vi "Uni final.vi"() -> ()   [LabVIEW 2025]
uses:
  <vilib>/MakerHub/LINX/Public/Peripherals/Analog/Analog Read 1 Chan.vi
  <vilib>/MakerHub/LINX/Public/Peripherals/Analog/Analog Read N Chans.vi
  <vilib>/MakerHub/LINX/Private/Local IO/LinxAnalogRead.vi
  <vilib>/MakerHub/LINX/Public/Utilities/Check Channel.vi
  <vilib>/MakerHub/LINX/Public/Utilities/Open Serial.vi
  <vilib>/MakerHub/LINX/Private/Utilties/Generate Error.vi
  <vilib>/MakerHub/LINX/LMH-LINX.lvlib
panel:
  out "Presión de Frenado":dbl(knob) scale=0.0..1000.0
  out "COLD":bool
  out "HOT":bool
  out "Presion de Frenado":dynamicdata(graph)
  out "Termometro K":dbl(slide) scale=0.0..400.0
  out "Termometro F":dbl(slide) scale=0.0..160.0
  out "Batería Descargada":bool
  out "Batería Cargada":bool
  in  "Serial Port":refnum<visa-resource-name>="N/A"
  in  "Stop":bool
  out "RPM":dbl(knob) scale=0.0..7000.0
  out "Batería":dbl(slide) scale=0.0..100.0
  out "Teermometro °C":dbl(slide) scale=0.0..170.0
  # "Universidad Politécnica Salesiana"
  # "PROYECTO 1"
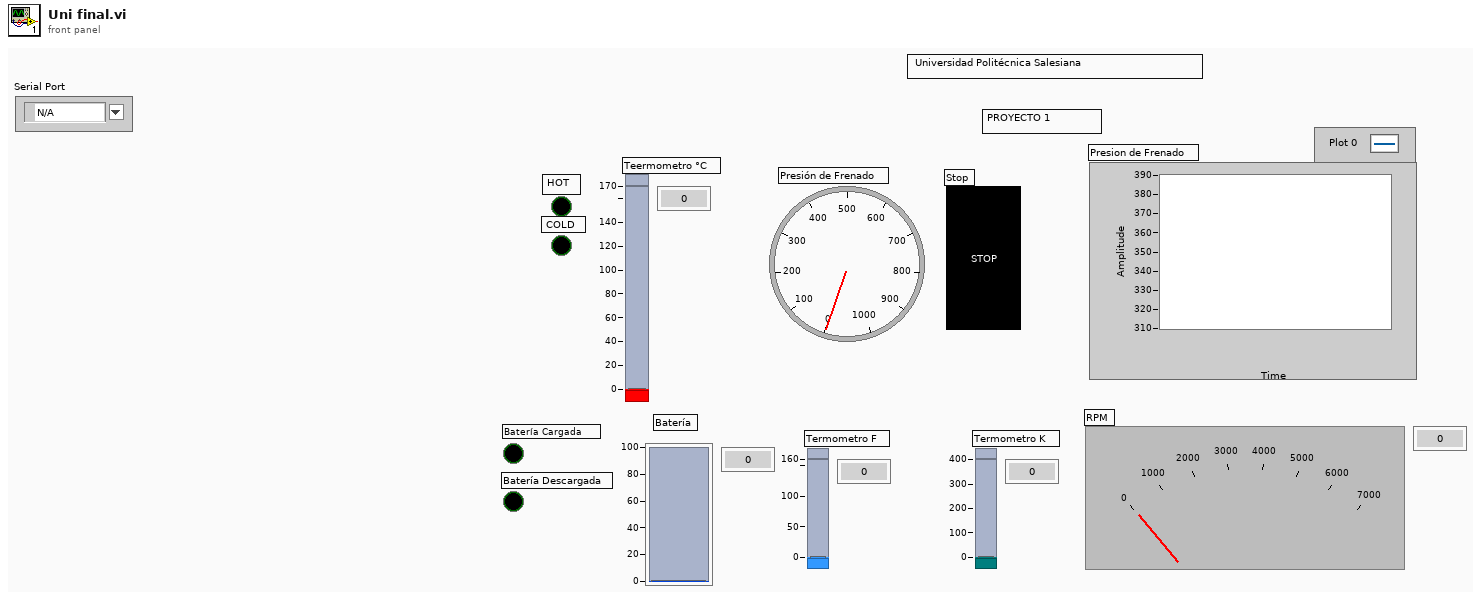
[diagram p1: front panel]
types:
  T1 = typedef "LMH-LINX.lvlib/LINX Ref.ctl" = cluster{"IO":T2, "Interface":T3, "LINX Device Config":T4}
  T2 = typedef "LMH-LINX.lvlib/Platform.ctl" = enum16{"Remote", "Local"}
  T3 = typedef "LMH-LINX.lvlib/Interface.ctl" = enum16{"Serial", "TCP"}
  T4 = typedef "LMH-LINX.lvlib/Device.lvlib/LINX Device Config.ctl" = cluster{"Interface":T3, "COM Port":refnum<visa-resource-name>, "TCP Configuration":T5, "Device Family":u8, "Device ID":u8, "Device Name":string, "TCP Ref":refnum<k5>, "Channels":T6}
  T5 = typedef "LMH-LINX.lvlib/Device.lvlib/TCP Config.ctl" = cluster{"IP Address":string, "Port":u16}
  T6 = typedef "LMH-LINX.lvlib/Channels.ctl" = cluster{"DI":u8[], "DO":u8[], "AI":u8[], "AO":u8[], "PWM":u8[], "QE":u8[], "UART":u8[], "I2C 2":u8[], "SPI":u8[], "CAN":u8[], "Servo":u8[], "AI Ref (V)":dbl, "AI Resolution (Bits)":u8, "AO Ref (V)":dbl, "AO Resolution (Bits)":u8}
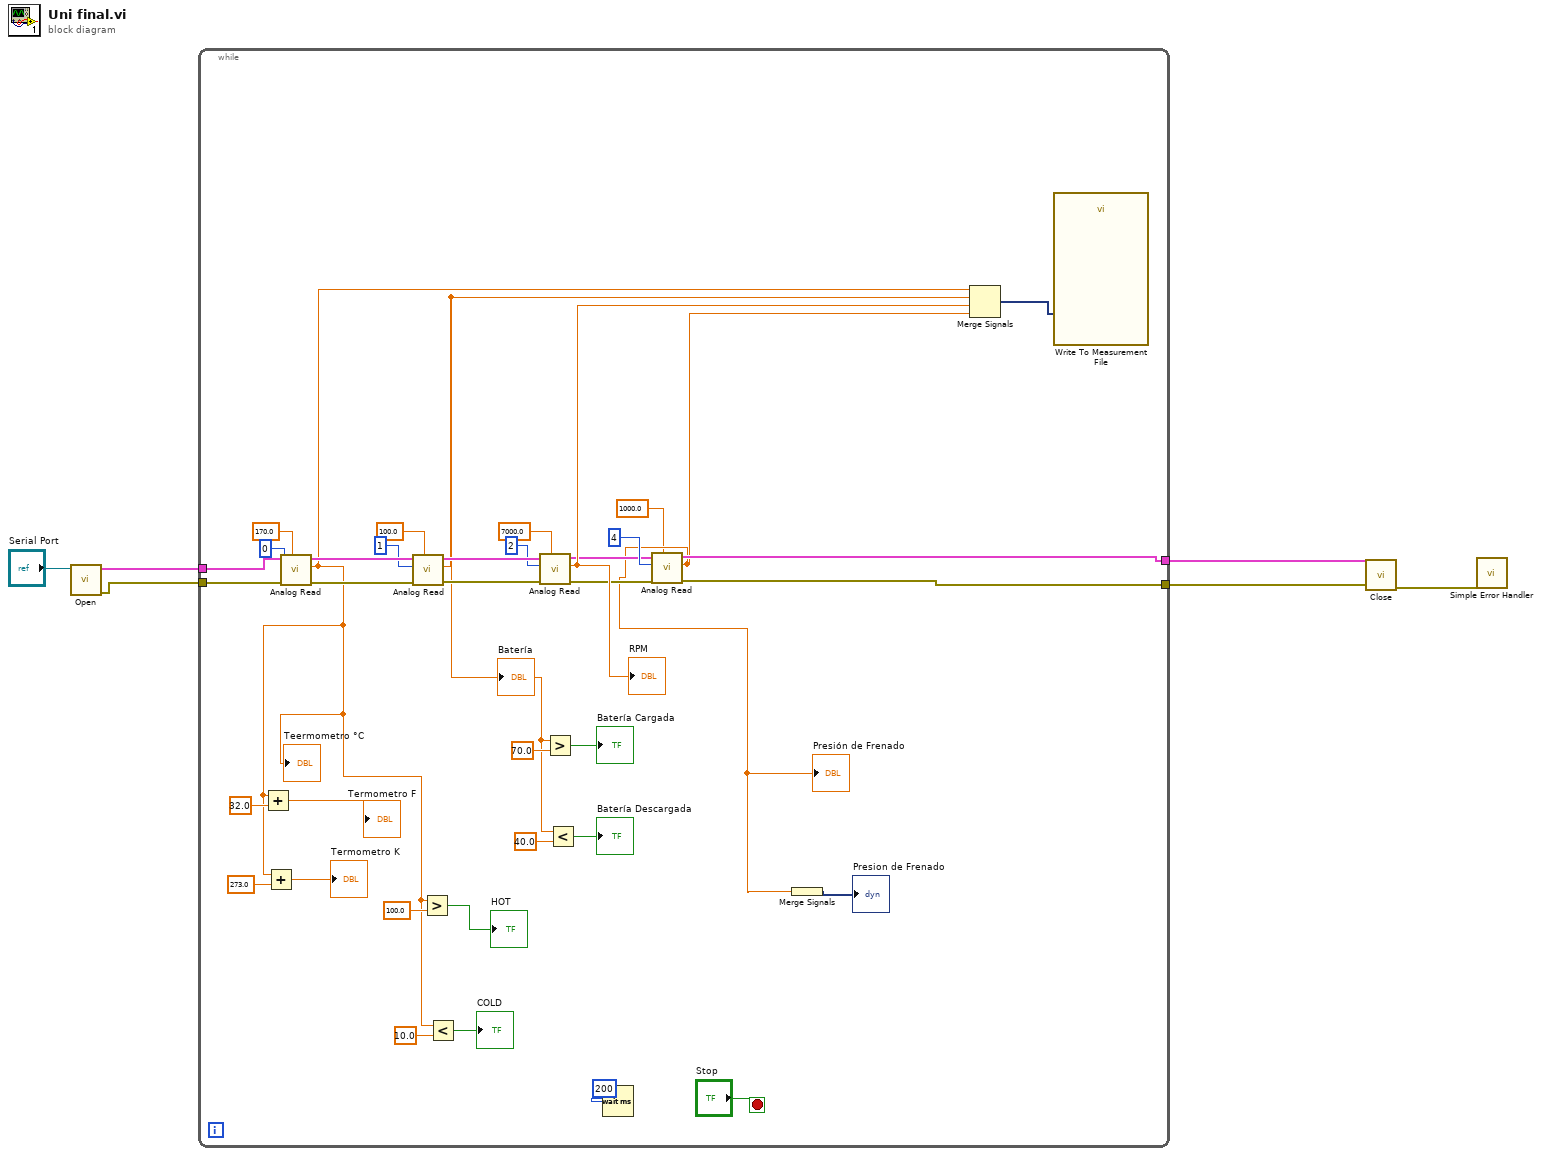
[diagram p0: block diagram]
diagram:
  n1 = call-poly <vilib>:"Open.vi"("Serial Port"="Serial Port") -> ("Error Out"=w4:errorcluster, "LINX Resource"=w5:T1)  [unwired: 8 in, 1 out]
  n2 = while {
    tunnel: w5 -> [w42]
    tunnel: w4 -> [w37]
    tunnel: [w10] -> w3
    tunnel: [w9] -> w2
    stop <- "Stop" stop-if-true
    n3 = call-poly <vilib>:"Analog Read.vi"("Analog Ref Override (V)"=170.0, "Error In"=w37, "Analog Channel"=u8 0, "LINX Resource"=w42) -> ("Error Out"=w38:errorcluster, "Voltage"=w15:dbl, "LINX Resource"=w41:T1)  [unwired: 4 in, 1 out]
    "Teermometro °C" <- w15
    n4 = Add(x=w15, y=32.0) -> (x+y=→"Termometro F":dbl)
    n5 = Add(x=w15, y=273.0) -> (x+y=→"Termometro K":dbl)
    n6 = call-poly <vilib>:"Analog Read.vi"("Analog Ref Override (V)"=100.0, "Error In"=w38, "Analog Channel"=u8 1, "LINX Resource"=w41) -> ("Error Out"=w39:errorcluster, "Voltage"=w20:dbl, "LINX Resource"=w40:T1)  [unwired: 4 in, 1 out]
    "Batería" <- w20
    n7 = Greater?(x=w15, y=100.0) -> (0:→"HOT":bool)
    n8 = Less?(x=w15, y=10.0) -> (x < y?=→"COLD":bool)
    n9 = call-poly <vilib>:"Analog Read.vi"("Analog Ref Override (V)"=7000.0, "Error In"=w39, "Analog Channel"=u8 2, "LINX Resource"=w40) -> ("Error Out"=w11:errorcluster, "Voltage"=w21:dbl, "LINX Resource"=w12:T1)  [unwired: 4 in, 1 out]
    "RPM" <- w21
    n10 = Greater?(x=w20, y=70.0) -> (0:→"Batería Cargada":bool)
    n11 = Less?(x=w20, y=40.0) -> (x < y?=→"Batería Descargada":bool)
    n12 = Wait (ms)(milliseconds to wait=u32 200) -> ()  [unwired: 1 out]
    n13 = call-poly <vilib>:"Analog Read.vi"("Analog Ref Override (V)"=1000.0, "Error In"=w11, "Analog Channel"=u8 4 ("DI Channel"), "LINX Resource"=w12) -> ("Error Out"=w9:errorcluster, "Voltage"=w8:dbl, "LINX Resource"=w10:T1)  [unwired: 4 in, 1 out]
    "Presión de Frenado" <- w8
    n14 = Merge Signals(w8) -> (→"Presion de Frenado":dynamicdata)
    n15 = Merge Signals(w15, w20, w21, w8) -> (w23:dynamicdata)
    n16 = call "Write To Measurement File"("Signals"=w23) -> ()  [unwired: 16 in, 3 out]
  }
  n17 = call <vilib>:"Close.vi"("Error In"=w2, "LINX Resource"=w3) -> ("Error Out"=w1:errorcluster)  [unwired: 9 in]
  n18 = call <vilib>:"Simple Error Handler.vi"("error in (no error)"=w1) -> ()  [unwired: 4 in, 5 out]
